vi "Identify.vi"(8 "error in (no error)":errorcluster, 11 "Skyworks Spur Test in":refnum<class "Skyworks Spur Test.lvclass">) -> (0 "error out":errorcluster, 2 "Plugin is Valid":bool, 3 "Skyworks Spur Test out":refnum<class "Skyworks Spur Test.lvclass">)   [LabVIEW 2018, in "Skyworks Spur Test.lvlib" / "Skyworks Spur Test.lvclass"]
uses:
  Skyworks Spur Test.lvclass
  C:/Sequence Automation/Plugins/Measurement Interface.lvlibp/Measurement Interface.lvclass
  Plugins/Measurement Interface.lvlibp/Private Methods/Measurement Definition Entry/Read Measurement Definition Entry.vi
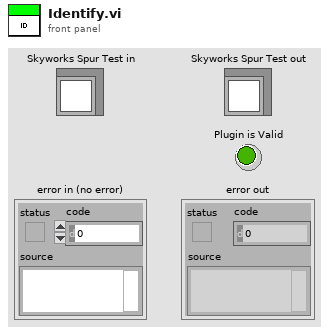
[diagram p1: front panel]
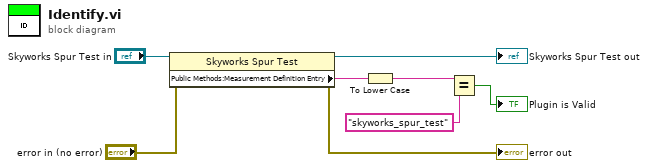
[diagram p0: block diagram]
diagram:
  n1 = property class="Skyworks Spur Test"(reference="Skyworks Spur Test in", error in="error in (no error)") -> (reference out=→"Skyworks Spur Test out":refnum<class "Skyworks Spur Test.lvclass">, error out=→"error out":errorcluster, "Public Methods:Measurement Definition Entry"=w4:string)
  n2 = To Lower Case(string=w4) -> (all lower case string=w3:string)
  n3 = Equal?(x=w3, y="skyworks_spur_test") -> (x = y?=→"Plugin is Valid":bool)
